vi "Stellengenauigkeit.vi"(7 "Genauigkeit (6)":i16, 11 "String":string) -> (0 "Formatstring":string, 3 "String out":string)   [LabVIEW 2020, in "Linearisierung v2.lvlib"]
uses:
  Linearisierung v2.lvlib
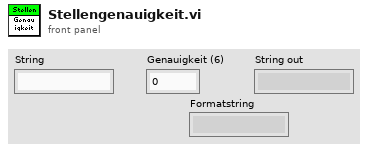
[diagram p1: front panel]
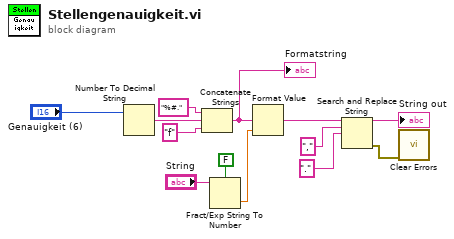
[diagram p0: block diagram]
diagram:
  n1 = Number To Decimal String(number="Genauigkeit (6)") -> (decimal integer string=w9:string)  [unwired: 1 in]
  n2 = Concatenate Strings("%#." ("Format-String"), w9, "f" ("Format-String")) -> (w7:string)
  "Formatstring" <- w7
  n3 = Fract/Exp String To Number(use system decimal point (T)=FALSE ("Systemdezimalzeichen verwenden (T)"), string="String") -> (number=w13:dbl)  [unwired: 2 in, 1 out]
  n4 = Format Value(format string=w7, value (0)=w13) -> (output string=w3:string)  [unwired: 1 in]
  n5 = Search and Replace String(input string=w3, search string="," ("Such-String"), replace string="." ("Ersetzungs-String (\"\")")) -> (result string=→"String out":string, error out=w1:errorcluster)  [unwired: 5 in, 2 out]
  n6 = call <vilib>:"Clear Errors.vi"("error in (no error)"=w1) -> ()  [unwired: 5 in, 2 out]
